vi "nominal channel unit.vi"(0 "channel":i32, 1 "is_present":bool, 5 "buf":string, 7 "cap":u32, 9 "out_needed":u32, 11 "error in (no error)":errorcluster) -> (3 "is_present out":bool, 4 "function return":i32, 6 "buf out":string, 10 "out_needed out":u32, 15 "error out":errorcluster)   [LabVIEW 2020, in "client.lvlib"]
doc: "int32_t nominal_channel_unit(int32_t channel,\n char *buf,\n uint32_t cap,\n uint32_t *out_needed,\n bool *is_present);"
uses:
  client.lvlib
  bin/nominalClient_64.dll
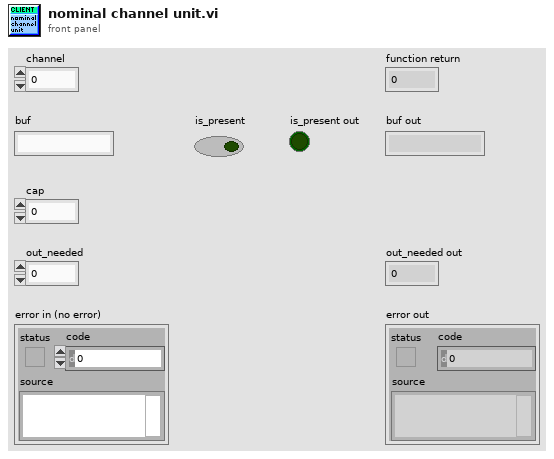
[diagram p1: front panel]
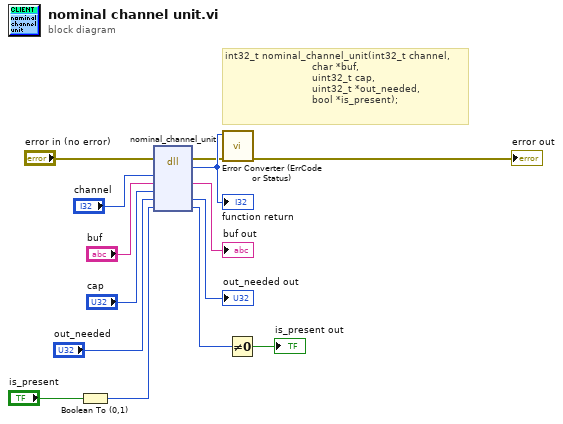
[diagram p0: block diagram]
diagram:
  # "int32_t nominal_channel_unit(int32_t channel,\n                             char *buf,\n                             uint32_t cap,\n                             uint32_t *out_needed,\n                             bool *is_present);"
  n1 = Boolean To (0,1)(Boolean="is_present") -> (0, 1=w6:i16)
  n2 = dll-call lib="C:/code/labview-client-rs/lv_src/bin/nominalClient_*.*" fn="nominal_channel_unit"(error in="error in (no error)", "channel"="channel", "buf"="buf", "cap"="cap", "out_needed"="out_needed", "is_present"=w6) -> (error out=w2:errorcluster, w14:i32, "buf"=→"buf out":string, "out_needed"=→"out_needed out":u32, "is_present"=w4:u8)  [unwired: 4 in, 1 out]
  "function return" <- w14
  n3 = call "Error Converter (ErrCode or Status).vi"("error in (no error)"=w2, "error code"=w14) -> ("error out"=→"error out":errorcluster)  [unwired: 9 in]
  n4 = Not Equal To 0?(x=w4) -> (x != 0?=→"is_present out":bool)
